vi "Dead Zone (DBL).vi"(2 "end of dead zone":dbl format="%.2f", 3 "start of dead zone":dbl format="%.2f", 4 "input point":dbl format="%.2f") -> (1 "output point":dbl format="%.2f")   [LabVIEW 2020, in "NI_AdvCtrl_nonlinear.lvlib"]
doc: "LabVIEW no longer supports this VI. You can obtain similar functionality by installing the LabVIEW Simulation Module.\n\nRealizes a region of zero output, the so-called dead zone. The output is zero, if the inequalities start of dead zone < input < end of dead zone hold true."
uses:
  <vilib>/addons/control/advanced/NI_AdvCtrl_nonlinear.lvlib
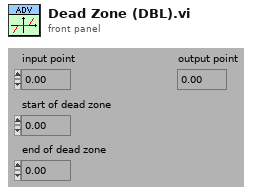
[diagram p1: front panel]
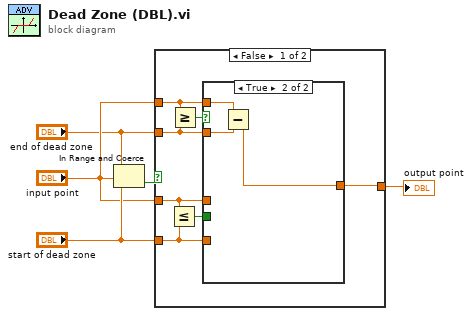
[diagram p0: block diagram]
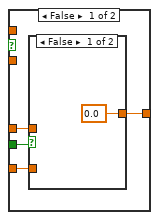
[diagram p2: hidden frame]
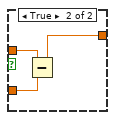
[diagram p3: hidden frame]
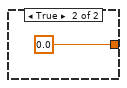
[diagram p4: hidden frame]
diagram:
  n1 = In Range and Coerce(upper limit="end of dead zone", x="input point", lower limit="start of dead zone") -> (In Range?=w1:bool)  [unwired: 1 out]
  n2 = case shown="False" w1 {
    tunnel: [w9 0.0] -> w2
    tunnel: "end of dead zone" -> [w10 _]
    tunnel: "input point" -> [w11 _]
    tunnel: "input point" -> [w7 _]
    tunnel: "start of dead zone" -> [w6 _]
    frame False {
      n3 = Less Or Equal?(x=w7, y=w6) -> (x <= y?=w8:bool)
      n4 = Greater Or Equal?(x=w11, y=w10) -> (x >= y?=w12:bool)
      n5 = case shown="True" w12 {
        tunnel: w11 -> [_ w23]
        tunnel: w10 -> [_ w22]
        tunnel: [w13 w21] -> w9
        tunnel: w8 -> [w16 _]
        tunnel: w7 -> [w15 _]
        tunnel: w6 -> [w14 _]
        frame False {
          n6 = case shown="False" w16 {
            tunnel: w15 -> [_ w20]
            tunnel: w14 -> [_ w19]
            tunnel: [0.0 w18] -> w13
            frame False {
            }
            frame True {
              n7 = Subtract(x=w20, y=w19) -> (x-y=w18:dbl)
            }
          }
        }
        frame True {
          n8 = Subtract(x=w23, y=w22) -> (x-y=w21:dbl)
        }
      }
    }
    frame True {
    }
  }
  "output point" <- w2
